vi "Carry out Monkey Activities.vi"(0 "Monkeys in":T1, 1 "#Rounds":i32, 2 "LCD":u64) -> (3 "Monkeys out":T1)   [LabVIEW 2020, in "AoC 2022.lvlib"]
uses:
  AoC 2022.lvlib
  Monkeys.ctl
  Monkey.ctl
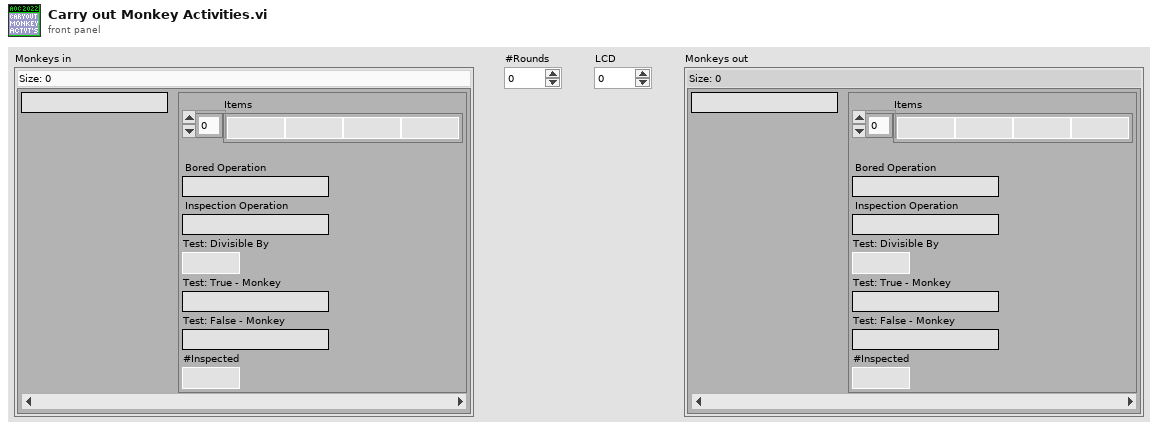
[diagram p1: front panel]
types:
  T1 = typedef "AoC 2022.lvlib/Monkeys.ctl" = map{string, T2}
  T2 = typedef "AoC 2022.lvlib/Monkey.ctl" = cluster{"Items":u64[], "Bored Operation":string, "Inspection Operation":string, "Test: Divisible By":u64, "Test: True - Monkey":string, "Test: False - Monkey":string, "#Inspected":i32}
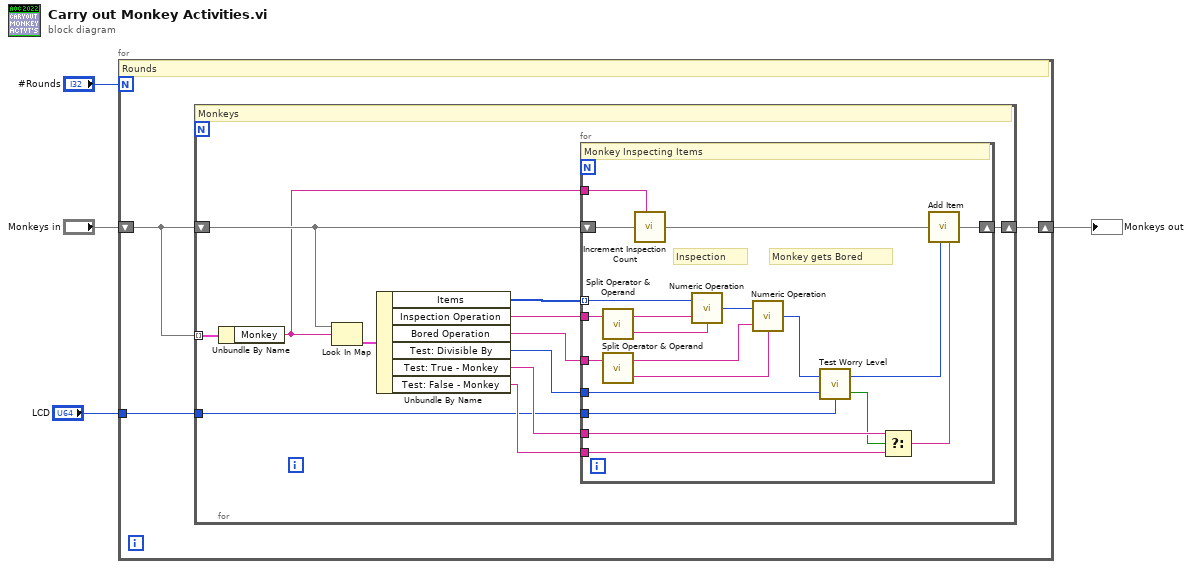
[diagram p0: block diagram]
diagram:
  n1 = for {
    N: "#Rounds" -> [_]
    shift-right: [w6] -> w4
    shift-left: "Monkeys in" -> [w7]
    tunnel: "LCD" -> [w5]
    # "Rounds"
    n2 = for {
      shift-right: [w19] -> w6
      shift-left: w7 -> [w12]
      tunnel: w7 -> [w10] mode=indexing
      tunnel: w5 -> [w8]
      # "Monkeys"
      n3 = Unbundle By Name(w10) -> ("Monkey"=w9:string)
      n4 = Look In Map(map=w12, key=w9) -> (value=w11:T2)  [unwired: 1 in, 1 out]
      n5 = Unbundle By Name(w11) -> ("Items"=w18:u64[], "Inspection Operation"=w17:string, "Bored Operation"=w16:string, "Test: Divisible By"=w15:u64, "Test: True - Monkey"=w14:string, "Test: False - Monkey"=w13:string)
      n6 = for {
        shift-right: [w39] -> w19
        shift-left: w12 -> [w27]
        tunnel: w18 -> [w24] mode=indexing
        tunnel: w17 -> [w38]
        tunnel: w16 -> [w35]
        tunnel: w15 -> [w23]
        tunnel: w14 -> [w31]
        tunnel: w13 -> [w30]
        tunnel: w9 -> [w25]
        tunnel: w8 -> [w22]
        # "Monkey gets Bored"
        # "Inspection"
        # "Monkey Inspecting Items"
        n7 = call "Split Operator & Operand.vi"("Operation"=w38) -> ("Operand"=w37:string, "Operator"=w36:string)  [unwired: 1 in]
        n8 = call "Split Operator & Operand.vi"("Operation"=w35) -> ("Operand"=w33:string, "Operator"=w32:string)  [unwired: 1 in]
        n9 = call "Increment Inspection Count.vi"("Monkeys in"=w27, "Monkey"=w25) -> ("Monkeys out"=w26:T1)  [unwired: 1 in]
        n10 = call "Numeric Operation.vi"("Operand 2"=w37, "Operator"=w36, "Operand 1"=w24) -> ("Result"=w34:u64)
        n11 = call "Numeric Operation.vi"("Operand 2"=w33, "Operator"=w32, "Operand 1"=w34) -> ("Result"=w21:u64)
        n12 = call "Test Worry Level.vi"("Test: Divisible By"=w23, "LCD"=w22, "Worry Level in"=w21) -> ("Test Result"=w29:bool, "Worry Level out"=w20:u64)  [unwired: 1 in]
        n13 = Select(t=w31, s=w29, f=w30) -> (s? t:f=w28:string)
        n14 = call "Add Item.vi"("Monkeys in"=w26, "Item"=w20, "Monkey"=w28) -> ("Monkeys out"=w39:T1)
      }
    }
  }
  "Monkeys out" <- w4
